vi "UnitTest_SelectData.vi"(8 "error in (no error)":errorcluster) -> (0 "error out":errorcluster)   [LabVIEW 2014, in "TableLogger_SQLite_Actor.lvlib" / "TableLogger_SQLite_Actor.lvclass"]
uses:
  TableLogger_SQLite_Actor.lvclass
  TableLogger_Actor/TableLoggerConfig.ctl
  TableLogger_Actor/TableLoggerTypes.ctl
  TableLogger_Actor/TableLoggerBackupConfig.ctl
  TableLogger_Actor/TableLogger_Actor.lvlib
  <vilib>/addons/_JKI Toolkits/Caraya/classes/Assert/Assert.lvclass
  <vilib>/addons/_JKI Toolkits/Caraya/classes/Test/Test.lvclass
panel:
  # "Please See the BlockDiagram for Select - Unit Test"
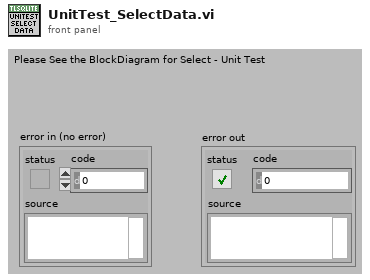
[diagram p1: front panel]
types:
  T1 = typedef "TableLogger_Actor.lvlib/TableLoggerConfig.ctl" = cluster{"TableLogger":T2, "DB File Path":path, "DB Backup Config":T3}
  T2 = typedef "TableLogger_Actor.lvlib/TableLoggerTypes.ctl" = enum16{"CSV Logger", "SQLite Logger"}
  T3 = typedef "TableLogger_Actor.lvlib/TableLoggerBackupConfig.ctl" = cluster{"Directory":path, "UTC Time Format":bool, "On Launch":bool, "Interval (Hours)":dbl, "Size Multiples (Bytes)":i32}
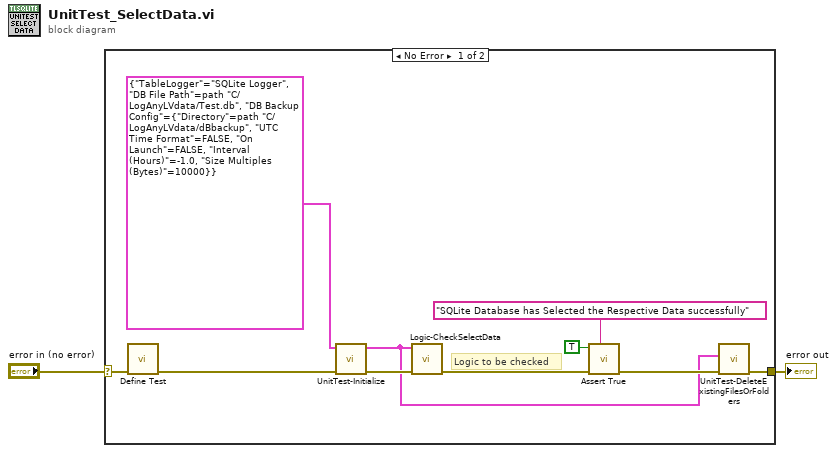
[diagram p0: block diagram]
diagram:
  n1 = case shown="No Error" "error in (no error)" {
    selector: "error in (no error)" -> [w4 w13]
    tunnel: [w5 w13] -> w2
    frame No Error {
      # "Logic to be checked"
      n2 = call <vilib>:"Define Test.vi"("error in (no error)"=w4) -> ("error out"=w11:errorcluster)  [unwired: 10 in]
      n3 = call "UnitTest-Initialize.vi"("error in"=w11, "Config IN"=T1 {"TableLogger"=enum."SQLite Logger", "DB File Path"=path "C:/LogAnyLVdata/Test.db", "DB Backup Config"={"Directory"=path "C:/LogAnyLVdata/dBbackup", "UTC Time Format"=FALSE, "On Launch"=FALSE, "Interval (Hours)"=-1.0, "Size Multiples (Bytes)"=10000}} ("TableLogger Config")) -> ("error out"=w10:errorcluster, "Config OUT"=w6:T1)  [unwired: 7 in, 1 out]
      n4 = call "Logic-CheckSelectData.vi"("error in (no error)"=w10, "TableLogger Config"=w6) -> ("error out"=w8:errorcluster)  [unwired: 9 in]
      n5 = call <vilib>:"Assert True.vi"("Label"="SQLite Database has Selected the Respective Data successfully", "error in (no error)"=w8, "True?"=TRUE) -> ("error out"=w7:errorcluster)  [unwired: 8 in]
      n6 = call "UnitTest-DeleteExistingFilesOrFolders.vi"("error in (no error)"=w7, "Config IN"=w6) -> ("error out"=w5:errorcluster)  [unwired: 9 in]
    }
    frame Error {
    }
  }
  "error out" <- w2
